vi "onInitialize.vi"(8 "error in (no error)":errorcluster, 11 "Artifactory in":refnum<class "Artifactory.lvclass">) -> (0 "error out":errorcluster, 3 "Artifactory out":refnum<class "Artifactory.lvclass">)   [LabVIEW 2021, in "Artifactory.lvclass"]
uses:
  Artifactory.lvclass
  Repository Event -- cluster.ctl
  Actions -- enum.ctl
  Artifactory.lvclass/Artifactory.ctl
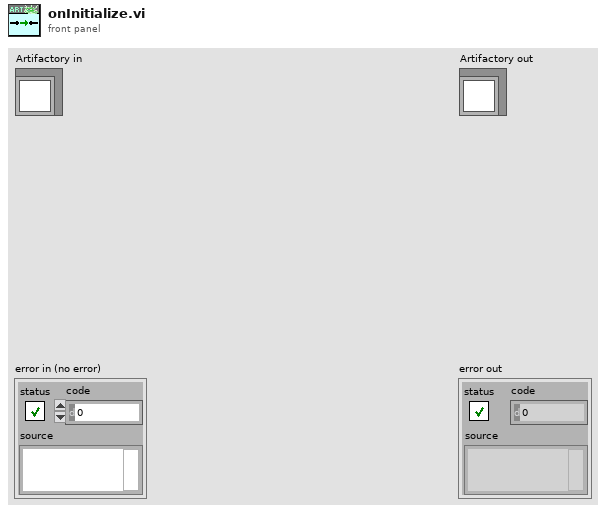
[diagram p1: front panel]
types:
  T1 = typedef "Artifactory.lvclass/Repository Event -- cluster.ctl" = cluster{"Action":T2, "Description":string}
  T2 = typedef "Artifactory.lvclass/Actions -- enum.ctl" = enum16{"Idle", "Custom Event", "Connecting to Artifactory", "Verifying Permissions", "Listing local repository", "Listing remote repository", "Computing changes", "Uploading file", "Downloading file"}
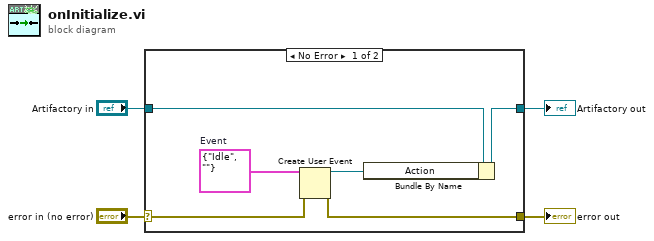
[diagram p0: block diagram]
diagram:
  n1 = case shown="No Error" "error in (no error)" {
    selector: "error in (no error)" -> [w6 w12]
    tunnel: [w5 w12] -> w3
    tunnel: [w8 w11] -> w1
    tunnel: "Artifactory in" -> [w7 w11]
    frame No Error {
      w10 = T1 {"Action"=enum."Idle", "Description"=""}  # Event
      n2 = Create User Event(user event datatype=w10, error in=w6) -> (user event=w9:refnum<user-event>, error out=w5:errorcluster)
      n3 = Bundle By Name(cluster=w7, "Action"=w9) -> (w8:refnum<class "Artifactory.lvclass">)
    }
    frame Error {
    }
  }
  "error out" <- w3
  "Artifactory out" <- w1
